vi "Check for Global Header.vi"(11 "Bytes in":u8[](array[numeric])) -> (1 "Offset":i32=-1, 2 "Global Header Present":bool, 3 "Bytes out":u8[](array[numeric]))   [LabVIEW 2021, in "pcap_Parse_Build_CIF.lvclass"]
doc: "Check if the global header is present by checking the first 8 bytes for magic number and version."
uses:
  pcap_Parse_Build_CIF.lvclass
  pcap_Parse_Build_CIF.lvclass/pcap_Parse_Build_CIF.ctl
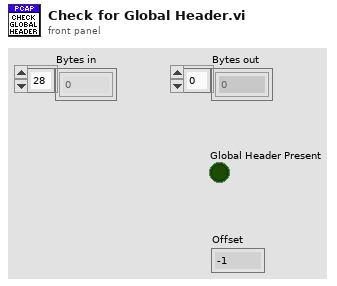
[diagram p1: front panel]
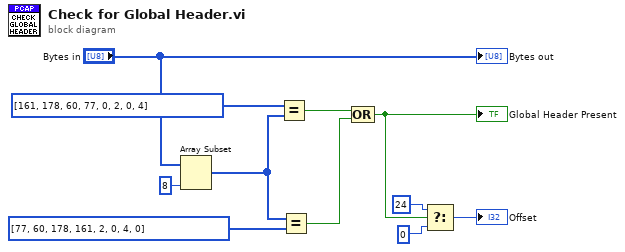
[diagram p0: block diagram]
diagram:
  n1 = Array Subset(array="Bytes in", length=8) -> (w7:u8[])  [unwired: 1 in]
  n2 = Equal?(x=u8[] [161, 178, 60, 77, 0, 2, 0, 4] ("unsigned byte array 2"), y=w7) -> (x = y?=w6:bool)
  n3 = Equal?(x=w7, y=u8[] [77, 60, 178, 161, 2, 0, 4, 0] ("unsigned byte array")) -> (x = y?=w5:bool)
  n4 = Compound Arithmetic op=OR(w6, w5) -> (w4:bool)
  "Global Header Present" <- w4
  n5 = Select(t=24 ("Offset"), s=w4, f=0 ("Offset")) -> (s? t:f=→"Offset":i32)
  "Bytes out" <- "Bytes in"
